vi "Cleanup.vi"(8 "error in (no error)":errorcluster, 11 "2DPanelBlank in":refnum<class "2DPanelBlank.lvclass">) -> (0 "error out":errorcluster)   [LabVIEW 2020, in "OOPanel.lvlib" / "2DPanelBlank.lvclass"]
uses:
  2DPanelBlank.lvclass
  ArrayPanel/ArrayPanel.lvclass
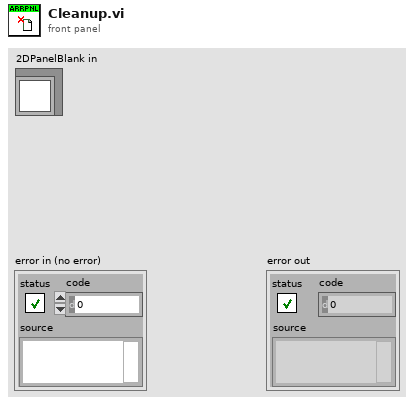
[diagram p1: front panel]
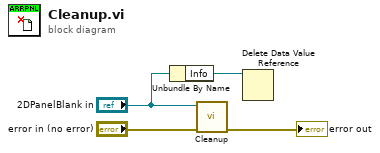
[diagram p0: block diagram]
diagram:
  n1 = Unbundle By Name("2DPanelBlank in") -> ("Info"=w1:refnum<data-value>)
  n2 = call-parent "Cleanup.vi"("error in (no error)"="error in (no error)", "ArrayPanel in"="2DPanelBlank in") -> ("error out"=→"error out":errorcluster)  [unwired: 9 in]
  n3 = Delete Data Value Reference(data value reference=w1) -> ()  [unwired: 1 in, 2 out]
